vi "旋转点（90）.vi"(11 "点":cluster{"x":i16, "y":i16}) -> (3 "点（90旋转）":cluster{"x":i16, "y":i16})   [LabVIEW 2012, in "Picture Box Tools.lvlib"]
uses:
  Picture Box Tools.lvlib
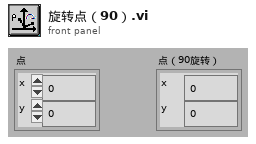
[diagram p1: front panel]
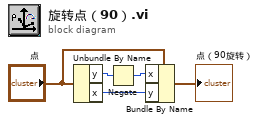
[diagram p0: block diagram]
diagram:
  n1 = Unbundle By Name("点") -> ("y"=w5:i16, "x"=w2:i16)
  n2 = Negate(x=w5) -> (-x=w4:i16)
  n3 = Bundle By Name(cluster="点", "x"=w4, "y"=w2) -> (→"点（90旋转）":cluster{"x":i16, "y":i16})
